vi "Example.vi"   [LabVIEW 2013]
uses:
  TSCAN Init.vi
  TSCAN ChannelCount.vi
  TSLIN ChannelCount.vi
  TSCAN SetMapping.vi
  TSCANFD SetMapping.vi
  TSLIN SetMapping.vi
  TSCAN Open.vi
  TSLIN Open.vi
  TSCAN Receive.vi
  TSCANFD Receive.vi
  TSlIN TransmitHeader&Receive.vi
  TSCANFD Transmit.vi
  TSLIN Transmit.vi
  TSCAN Transmit.vi
  TSCAN Close.vi
  TSCAN LoadDBC.vi
  TSCAN Dll.vi
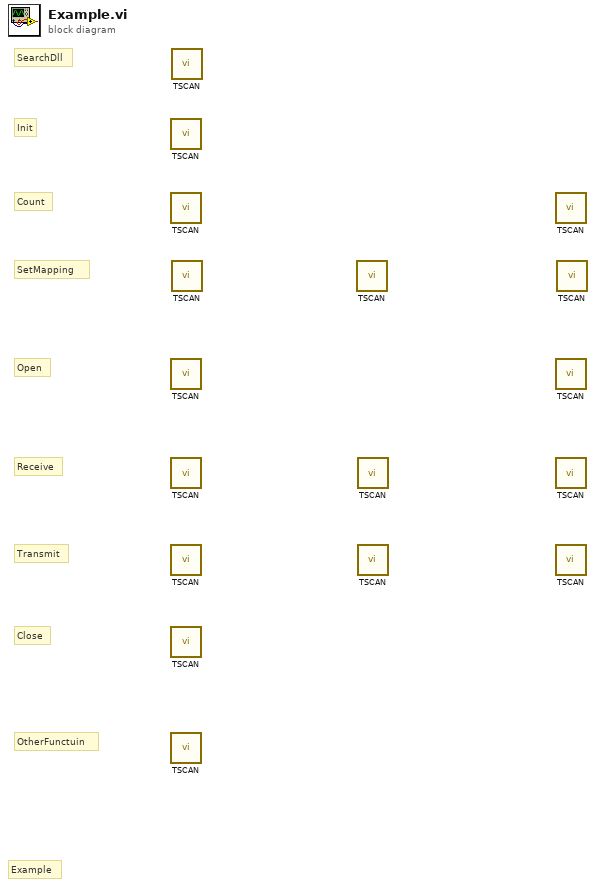
[diagram p0: block diagram]
diagram:
  # "Example"
  # "OtherFunctuin"
  # "SearchDll"
  # "Count"
  # "Close"
  # "Transmit"
  # "Receive"
  # "Open"
  # "SetMapping"
  # "Init"
  n1 = call-poly "TSCAN.vi"() -> ()  [unwired: 14 in, 2 out]
  n2 = call-poly "TSCAN.vi"() -> ()  [unwired: 13 in, 3 out]
  n3 = call-poly "TSCAN.vi"() -> ()  [unwired: 13 in, 3 out]
  n4 = call-poly "TSCAN.vi"() -> ()  [unwired: 13 in, 3 out]
  n5 = call-poly "TSCAN.vi"() -> ()  [unwired: 14 in, 2 out]
  n6 = call-poly "TSCAN.vi"() -> ()  [unwired: 14 in, 2 out]
  n7 = call-poly "TSCAN.vi"() -> ()  [unwired: 12 in, 4 out]
  n8 = call-poly "TSCAN.vi"() -> ()  [unwired: 15 in, 1 out]
  n9 = call-poly "TSCAN.vi"() -> ()  [unwired: 14 in, 2 out]
  n10 = call-poly "TSCAN.vi"() -> ()  [unwired: 13 in, 3 out]
  n11 = call-poly "TSCAN.vi"() -> ()  [unwired: 13 in, 3 out]
  n12 = call-poly "TSCAN.vi"() -> ()  [unwired: 14 in, 2 out]
  n13 = call-poly "TSCAN.vi"() -> ()  [unwired: 14 in, 2 out]
  n14 = call-poly "TSCAN.vi"() -> ()  [unwired: 13 in, 3 out]
  n15 = call-poly "TSCAN.vi"() -> ()  [unwired: 14 in, 2 out]
  n16 = call-poly "TSCAN.vi"() -> ()  [unwired: 14 in, 2 out]
  n17 = call-poly "TSCAN.vi"() -> ()  [unwired: 13 in, 3 out]
